vi "picoquant_make_new_dataset.vi"(8 "error in (no error)":errorcluster, 10 "dataset_path":string, 11 "picoharp in":refnum<class "picoharp.lvclass">) -> (0 "error out":errorcluster, 3 "picoharp out":refnum<class "picoharp.lvclass">)   [LabVIEW 2015, in "picoharp.lvclass"]
uses:
  picoharp.lvclass
  picoharp.lvclass/picoharp.ctl
  Data Logger Class/data_logger.lvclass
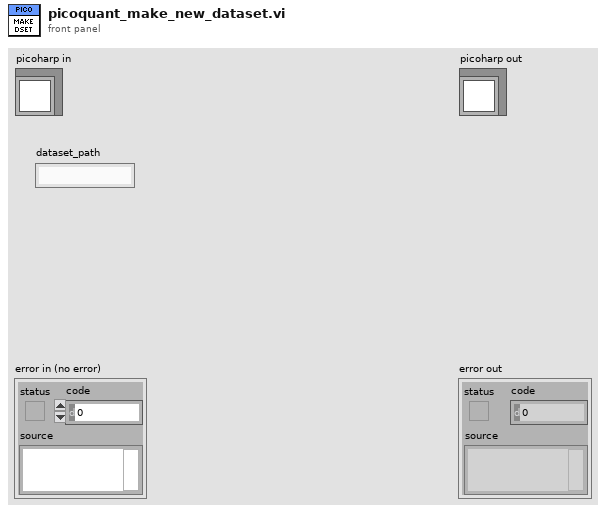
[diagram p1: front panel]
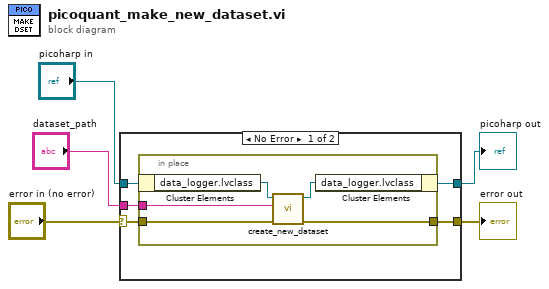
[diagram p0: block diagram]
diagram:
  n1 = case shown="No Error" "error in (no error)" {
    selector: "error in (no error)" -> [w7 w16]
    tunnel: "dataset_path" -> [w9 _]
    tunnel: "picoharp in" -> [w10 w17]
    tunnel: [w8 w17] -> w2
    tunnel: [w6 w16] -> w1
    frame No Error {
      n2 = in-place {
        in-place-border: w9 -> [w14]
        in-place-border: w7 -> [w12]
        in-place-border: [w11] -> w6
        n3 = in-place-cluster #1(w10) -> ("data_logger.lvclass"=w15:refnum<class "data_logger.lvclass">)
        n4 = call-dynamic "create_new_dataset.vi"("error in (no error)"=w12, "Path"=w14, "data_logger in"=w15) -> ("error out"=w11:errorcluster, "data_logger out"=w13:refnum<class "data_logger.lvclass">)  [unwired: 7 in]
        n5 = in-place-cluster #1("data_logger.lvclass"=w13) -> (w8:refnum<class "picoharp.lvclass">)
      }
    }
    frame Error {
    }
  }
  "error out" <- w1
  "picoharp out" <- w2
